vi "Set LabPython Server Path.vi"() -> ()   [LabVIEW 2011]
panel:
  in  "path (empty: python24.dll)":path=path "C:/Data/Antonio/software/WinPython-32bit-2.7.5.3/python-2.7.5/python27.dll"
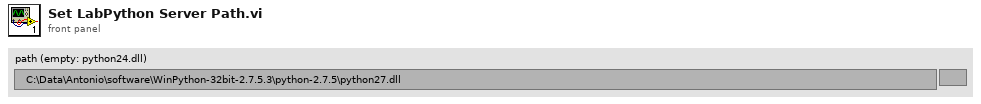
[diagram p1: front panel]
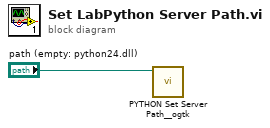
[diagram p0: block diagram]
diagram:
  n1 = call <userlib>:"PYTHON Set Server Path__ogtk.vi"("path (empty: python24.dll)"="path (empty: python24.dll)") -> ()  [unwired: 6 in, 1 out]
